vi "AIP Read Depth Min.vi"(8 "error in (no error)":errorcluster, 11 "AIP Instrument in":refnum<class "AIP Instrument.lvclass">) -> (0 "error out":errorcluster, 2 "Depth":dbl, 3 "AIP Instrument out":refnum<class "AIP Instrument.lvclass">)   [LabVIEW 2015, in "AIP Instrument.lvlib" / "AIP Instrument.lvclass"]
uses:
  AIP Instrument.lvclass
  AIP Instrument.lvclass/AIP Instrument.ctl
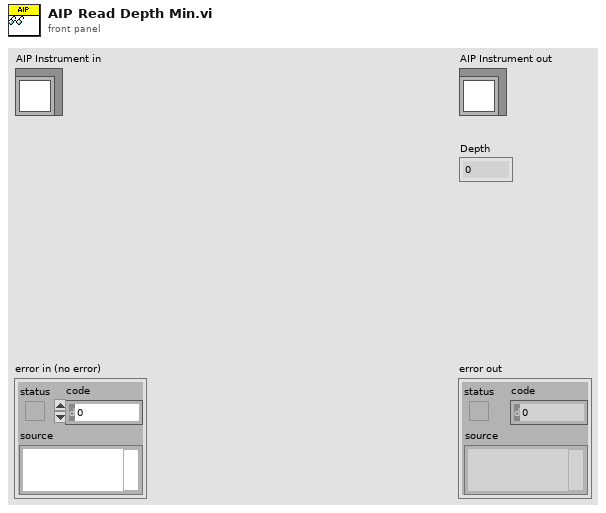
[diagram p1: front panel]
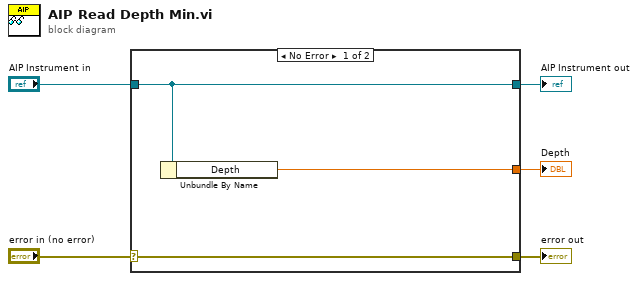
[diagram p0: block diagram]
diagram:
  n1 = case shown="No Error" "error in (no error)" {
    selector: "error in (no error)" -> [w8 w9]
    tunnel: [w8 w9] -> w4
    tunnel: [w7 w10] -> w2
    tunnel: "AIP Instrument in" -> [w7 w10]
    tunnel: [w6 _] -> w1
    frame No Error {
      n2 = Unbundle By Name(w7) -> ("Depth"=w6:sgl)
    }
    frame Error {
    }
  }
  "error out" <- w4
  "AIP Instrument out" <- w2
  "Depth" <- w1
